vi "meTEC_Create Error Cluster (Monitoring Loop).vi"(8 "error in (no error)":errorcluster, 9 "Error Parameter":string, 10 "Error Instance":string, 11 "Error Number":string) -> (0 "error out":errorcluster)   [LabVIEW 2023]
panel:
  # "--- Outputs ---"
  # "--- Inputs ---"
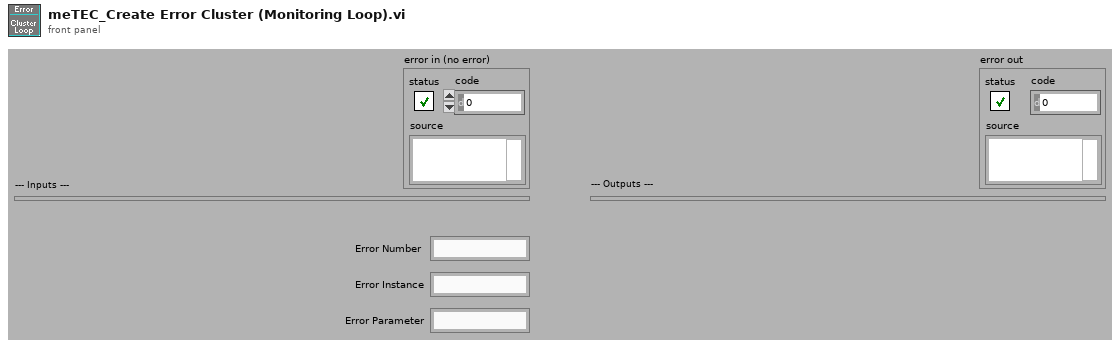
[diagram p1: front panel]
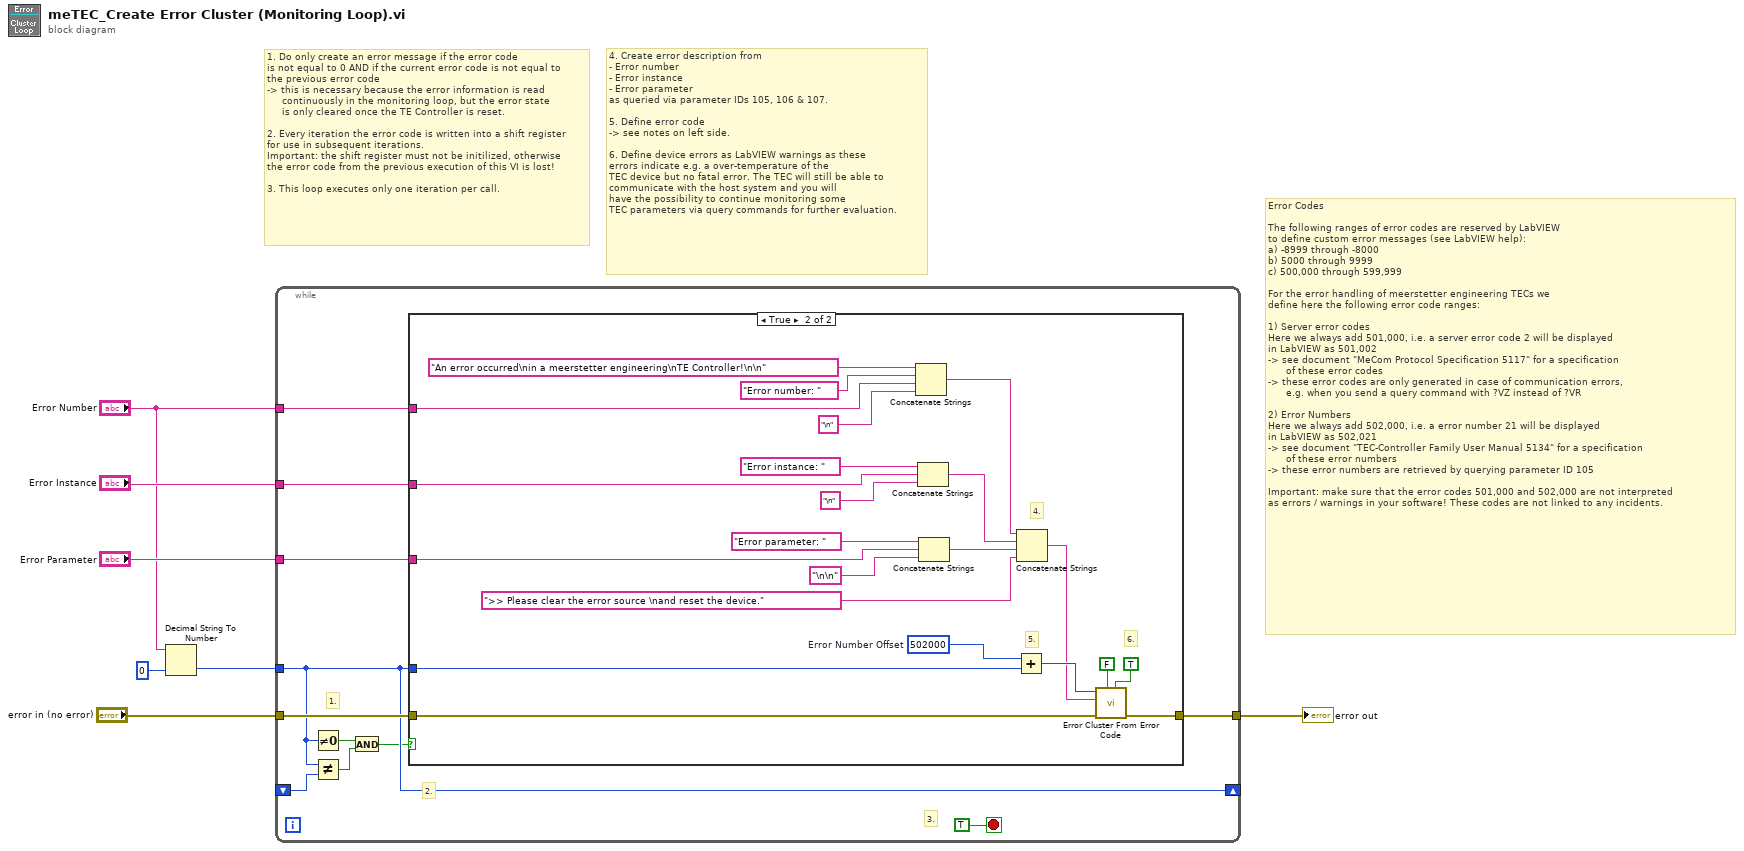
[diagram p0: block diagram]
diagram:
  # "1. Do only create an error message if the error code\nis not equal to 0 AND if the current error code is not equal to \nthe previous error code\n-> this is necessary because the error information is read\n     continuously in the monitoring loop, but the error state\n     is only cleared once the TE Controller is reset. \n\n2. Every iteration the error code is written into a shift register\nfor use in subsequent iterations.\nImportant: the shift register must not be initilized, otherwise\nthe error code from the previous execution of this VI is lost!\n\n3. This loop executes only one iteration per call."
  # "Error Codes\n\nThe following ranges of error codes are reserved by LabVIEW\nto define custom error messages (see LabVIEW help):\na) -8999 through -8000 \nb) 5000 through 9999 \nc) 500,000 through 599,999\n\nFor the error handling of meerstetter engineering TECs we\ndefine here the following error code ranges:\n\n1) Server error codes\nHere we always add 501,000, i.e. a server error code 2 will be displayed\nin LabVIEW as 501,002\n-> see document \"MeCom Protocol Specification 5117\" for a specification \n      of these error codes\n-> these error codes are only generated in case of communication errors, \n      e.g. when you send a query command with ?VZ instead of ?VR \n\n2) Error Numbers\nHere we always add 502,000, i.e. a error number 21 will be displayed\nin LabVIEW as 502,021 \n-> see document \"TEC-Controller Family User Manual 5134\" for a specification \n      of these error numbers\n-> these error numbers are retrieved by querying parameter ID 105 \n\nImportant: make sure that the error codes 501,000 and 502,000 are not interpreted\nas errors / warnings in your software! These codes are not linked to any incidents."
  # "4. Create error description from\n- Error number\n- Error instance\n- Error parameter\nas queried via parameter IDs 105, 106 & 107.\n\n5. Define error code\n-> see notes on left side.\n\n6. Define device errors as LabVIEW warnings as these\nerrors indicate e.g. a over-temperature of the \nTEC device but no fatal error. The TEC will still be able to \ncommunicate with the host system and you will \nhave the possibility to continue monitoring some \nTEC parameters via query commands for further evaluation."
  n1 = Decimal String To Number(string="Error Number", default (0L)=0 ("default (0 U32)")) -> (number=w1:i32)  [unwired: 1 in, 1 out]
  n2 = while {
    tunnel: [w18] -> w7
    tunnel: "error in (no error)" -> [w17]
    tunnel: "Error Parameter" -> [w16]
    tunnel: "Error Instance" -> [w15]
    tunnel: "Error Number" -> [w14]
    tunnel: w1 -> [w12]
    shift-right: [w12] -> _
    shift-left: _ -> [w13]
    stop <- TRUE stop-if-true
    # "3."
    # "1."
    # "2."
    n3 = Not Equal To 0?(x=w12) -> (x != 0?=w11:bool)
    n4 = Not Equal?(x=w12, y=w13) -> (x != y?=w10:bool)
    n5 = And(x=w11, y=w10) -> (x .and. y?=w9:bool)
    n6 = case shown="True" w9 {
      tunnel: [w19 w27] -> w18
      tunnel: w17 -> [w19 w26]
      tunnel: w16 -> [_ w25]
      tunnel: w15 -> [_ w24]
      tunnel: w14 -> [_ w23]
      tunnel: w12 -> [_ w21]
      frame False {
      }
      frame True {
        w28 = 502000  # Error Number Offset
        # "6."
        # "5."
        # "4."
        n7 = Concatenate Strings("An error occurred\nin a meerstetter engineering\nTE Controller!\n\n" ("string"), "Error number: " ("string"), w23, "\n" ("string")) -> (w30:string)
        n8 = Concatenate Strings("Error instance: " ("string"), w24, "\n" ("string")) -> (w31:string)
        n9 = Concatenate Strings("Error parameter: " ("string"), w25, "\n\n" ("string")) -> (w32:string)
        n10 = Add(x=w28, y=w21) -> (x+y=w40:i32)
        n11 = Concatenate Strings(w30, w31, w32, ">> Please clear the error source \nand reset the device." ("string")) -> (w29:string)
        n12 = call <vilib>:"Error Cluster From Error Code.vi"("is warning? (False)"=TRUE, "show call chain? (False)"=FALSE, "error in (no error)"=w26, "error message (\"\")"=w29, "error code (0)"=w40) -> ("error out"=w27:errorcluster)  [unwired: 4 in]
      }
    }
  }
  "error out" <- w7
